vi "DalsaFalcon2TLCMode.vi"() -> ()   [LabVIEW 2011]
panel:
  in  "Set TLC?":bool=TRUE
  out "String Read 2":string
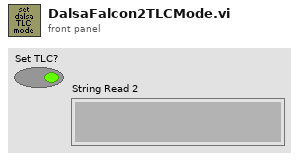
[diagram p1: front panel]
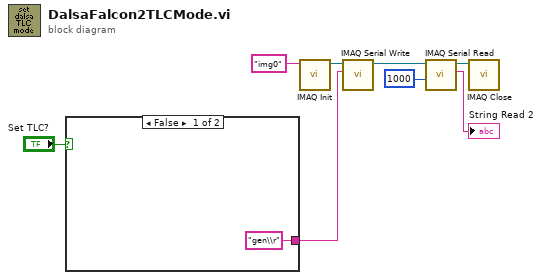
[diagram p0: block diagram]
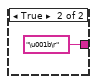
[diagram p2: hidden frame]
diagram:
  n1 = case shown="False" "Set TLC?" {
    tunnel: ["gen\\r" ("String to write") "\u001b\r" ("String to write")] -> w6
    frame False {
    }
    frame True {
    }
  }
  n2 = call <vilib>:"IMAQ Init.vi"("Interface Name"="img0") -> ("IMAQ Session Out"=w7:refnum<k11>)  [unwired: 9 in, 1 out]
  n3 = call <vilib>:"IMAQ Serial Write.vi"("String to write"=w6, "IMAQ Session In"=w7) -> ("IMAQ Session Out"=w3:refnum<k11>)  [unwired: 2 in, 5 out]
  n4 = call <vilib>:"IMAQ Serial Read.vi"("Timeout"=u32 1000, "IMAQ Session In"=w3) -> ("String Read"=→"String Read 2":string, "IMAQ Session Out"=w2:refnum<k11>)  [unwired: 4 in, 2 out]
  n5 = call <vilib>:"IMAQ Close.vi"("IMAQ Session In"=w2) -> ()  [unwired: 10 in, 1 out]
